vi "Just video2.vi"() -> ()   [LabVIEW 2014]
uses:
  <vilib>/Platform/TimedLoop/XDataNode/wakeup.ctl
  <vilib>/Platform/TimedLoop/XDataNode/XDNodeRunTimeDep.lvlib
  <vilib>/Platform/TimedLoop/XDataNode/nitl_modes.ctl
  <vilib>/Platform/TimedLoop/XDataNode/timing_clust.ctl
  <vilib>/Platform/TimedLoop/XDataNode/XDataNode.xnode
  <vilib>/vision/Avi1.llb/AviRefnum.ctl
panel:
  in  "Image Index":dbl=1.0 min=1.0
  in  "Capture and Save Image":bool
  in  "Averaging":bool
  in  "Reset Averaging":bool
  in  "Capture Video":bool
  out "Image":u32[][](graph)
  in  "New Video File":bool
  in  "Video Index":dbl=1.0 min=1.0 step=1.0
  out "Path Out":path
  in  "Video Capture Rate (Hz)":dbl=30.0
  in  "Stop All":bool
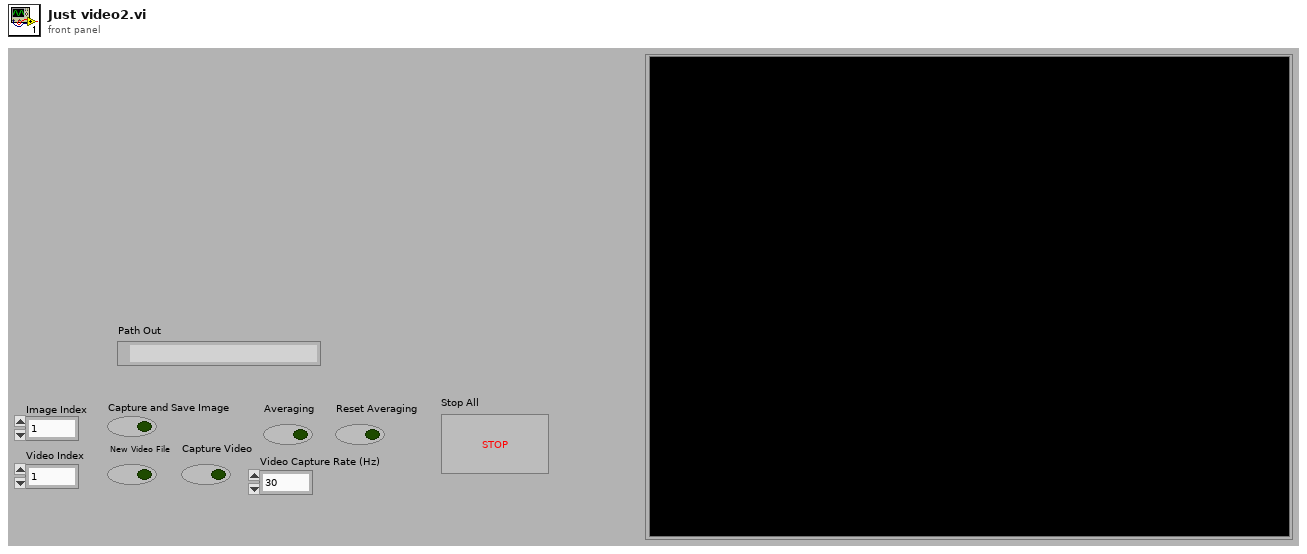
[diagram p1: front panel]
types:
  T1 = enum32{"setting", "request", "request control", "info", "statistics", "system settings", "I/O sub system", "HRT control", "camera descriptions", "device specific data", "event sub system settings", "event sub system results", "image memory manager"}
  T2 = typedef "AviRefnum.ctl" = refnum<k1>
  T3 = typedef "XDNodeRunTimeDep.lvlib/timing_clust.ctl" = cluster{"Expected End [f-1]":u64, "Actual End [f-1]":u64, "Finished Late? [f-1]":bool, "Expected End [i-1]":u64, "Actual End [i-1]":u64, "Finished Late? [i-1]":bool, "Expected Start [i]":u64, "Actual Start [i]":u64, "Expected Start [f]":u64, "Actual Start [f]":u64, "Source Name":string, "Structure Name":string, "Period":i64, "Deadline":i64, "Offset":i64, "Start":i64, "Priority":i32, "Timeout":i32, "Mode":T4, "Wakeup Reason":T5, "Error":errorcluster, "Source Type":string, "Secondary Source Type":string, "Global End Time":u64, "Global Start Time":u64, "Frame Duration":u64, "Iteration Duration":u64, "Assigned CPU":i32, "I/O Scan Engine Mode":u32}
  T4 = typedef "XDNodeRunTimeDep.lvlib/nitl_modes.ctl" = enum32{"No Change", "Process missed periods, maintain original phase", "Discard missed periods, maintain original phase", "Process missed periods, ignore original phase", "Discard missed periods, ignore original phase"}
  T5 = typedef "XDNodeRunTimeDep.lvlib/wakeup.ctl" = enum32{"Normal", "Aborted", "Asynchronous wakeup", "Timing source error", "Timed loop error", "Timeout"}
  T6 = typedef "Image Type" = u32
  T7 = typedef "IMAQ Image.ctl" = refnum<image>
  T8 = typedef "imagedata.ctl" = cluster{"image type":i32, "image depth":i32, "image":u8[], "mask":u8[], "colors":u32[], "Rectangle":cluster{"left":i16, "top":i16, "right":i16, "bottom":i16}}
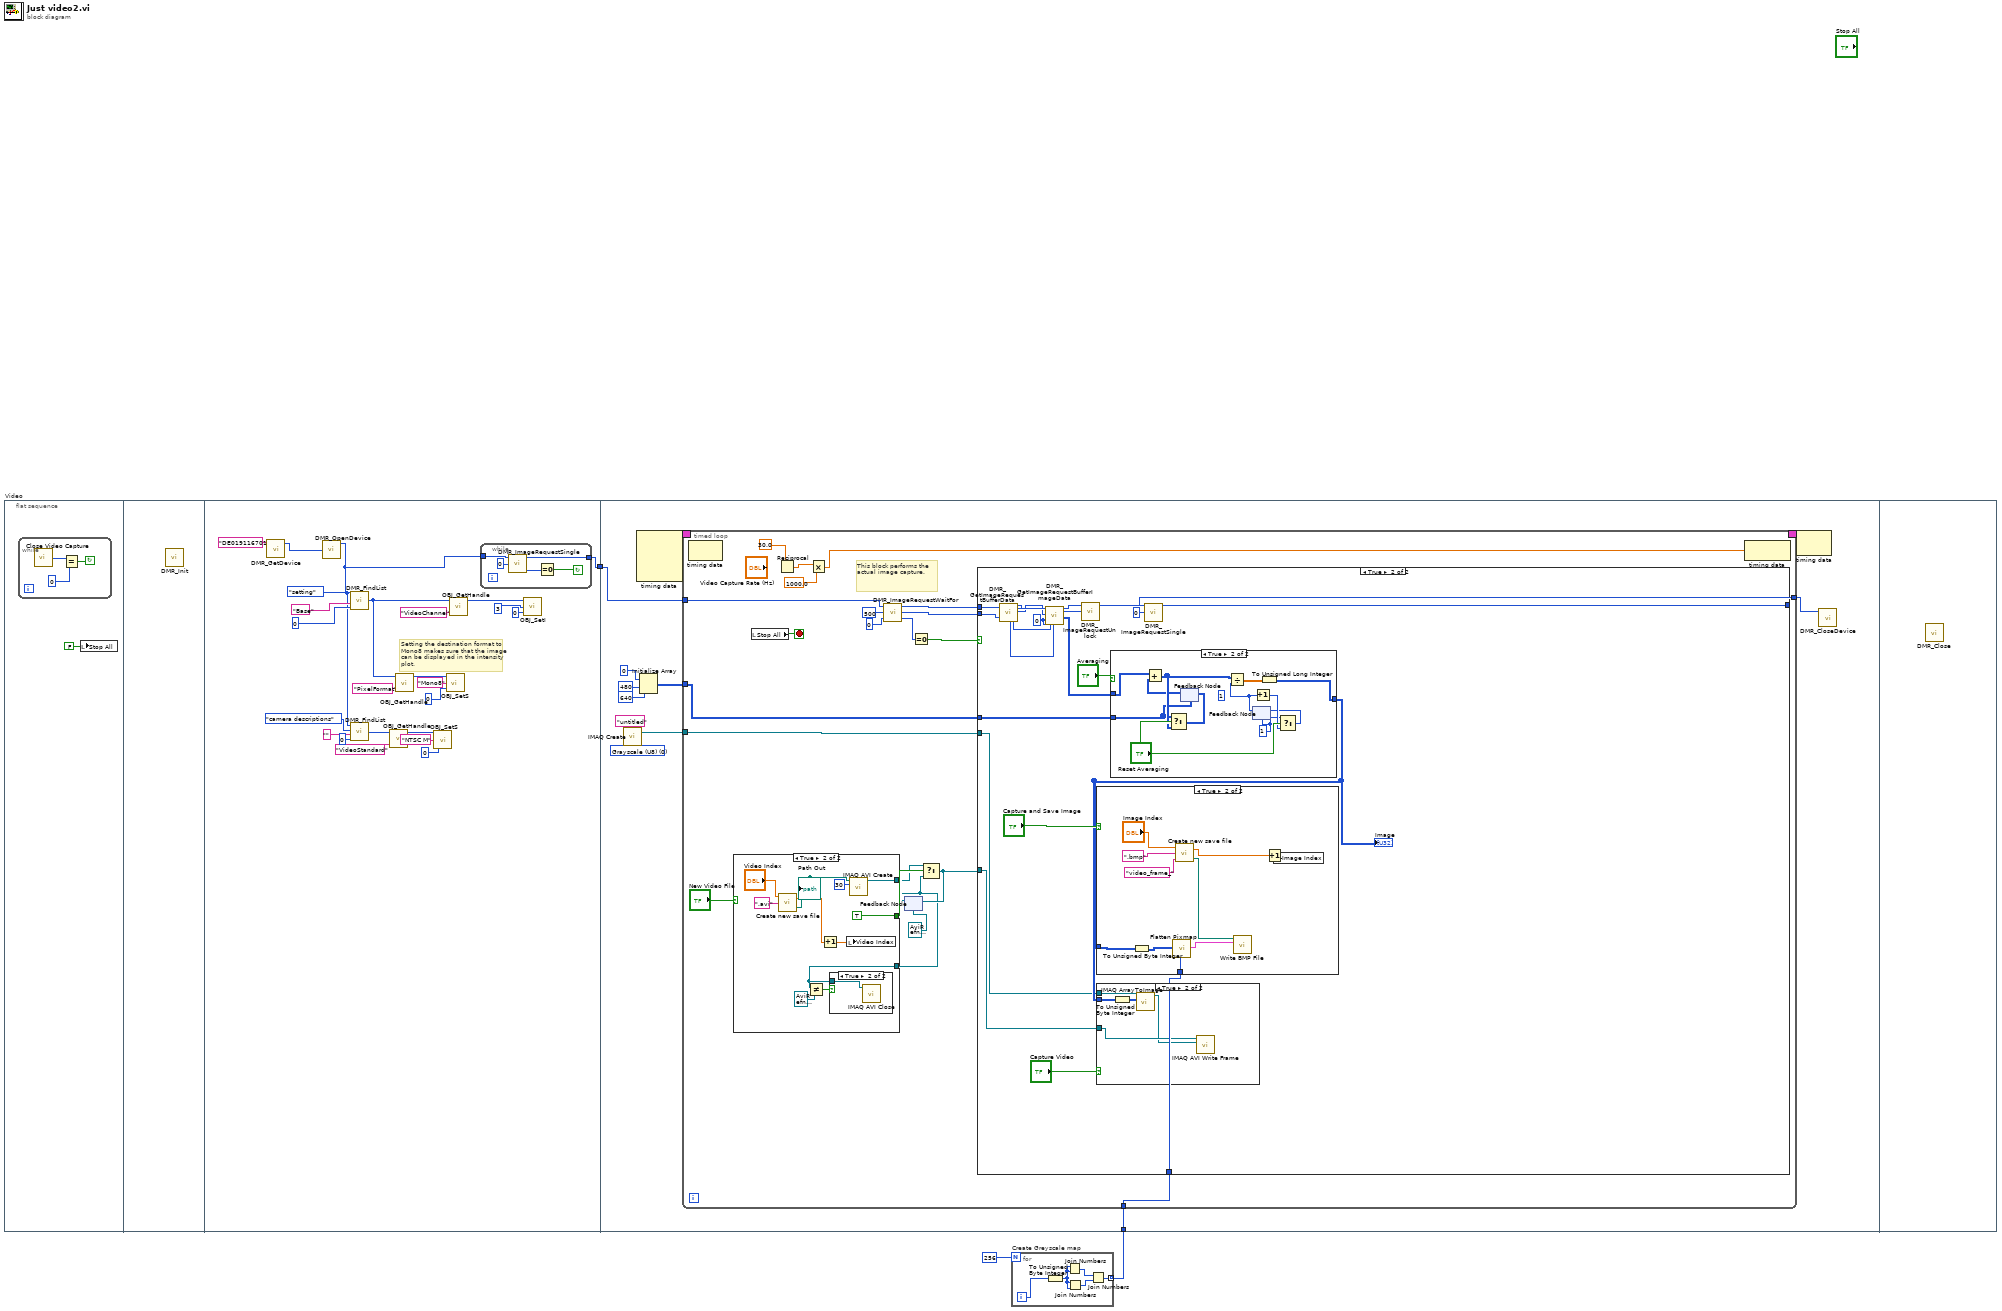
[diagram p0: block diagram]
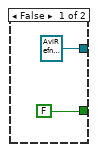
[diagram p2: hidden frame]
diagram:
  n1 = flat-sequence "Video" {
    tunnel: [w12] -> w3
    tunnel: w3 -> [w48]
    tunnel: w1 -> [w46]
    frame #0 {
      n2 = while {
        stop <- w5 continue-if-true
        n3 = call "Close Video Capture.vi"() -> ("error code OUT"=w7:i32)
        n4 = Equal?(x=w7, y=0) -> (x = y?=w5:bool)
      }
      n5 = local write "Stop All"(FALSE ("Stop All")) -> ()
    }
    frame #1 {
      n6 = call "DMR_Init.vi"() -> ()  [unwired: 3 out]
    }
    frame #2 {
      # "Setting the destination format to Mono8 makes sure that the image can be displayed in the intensity plot."
      n7 = call "DMR_GetDevice.vi"("search string IN"="DE019116701") -> ("device handle OUT"=w30:i32)  [unwired: 4 in, 2 out]
      n8 = call "DMR_OpenDevice.vi"("device handle IN"=w30) -> ("driver handle OUT"=w13:i32)  [unwired: 4 out]
      n9 = call "DMR_FindList.vi"("flags IN"=u32 0 ("flags"), "list name IN"="" ("String"), "list type IN"=T1."camera descriptions", "driver handle IN"=w13) -> ("list handle OUT"=w16:i32)  [unwired: 2 out]
      n10 = call "DMR_FindList.vi"("flags IN"=u32 0 ("flags"), "list name IN"="Base", "list type IN"=T1."setting", "driver handle IN"=w13) -> ("list handle OUT"=w14:i32)  [unwired: 2 out]
      n11 = call "OBJ_GetHandle.vi"("object name IN"="VideoStandard", "list handle IN"=w16) -> ("object handle OUT"=w10:i32)  [unwired: 3 out]
      n12 = call "OBJ_GetHandle.vi"("object name IN"="PixelFormat", "list handle IN"=w14) -> ("object handle OUT"=w24:i32)  [unwired: 3 out]
      n13 = call "OBJ_SetS.vi"("value index IN"=0, "value IN"="NTSC M", "object handle IN"=w10) -> ()  [unwired: 2 out]
      n14 = call "OBJ_SetS.vi"("value index IN"=0, "value IN"="Mono8" ("value"), "object handle IN"=w24) -> ()  [unwired: 2 out]
      n15 = call "OBJ_GetHandle.vi"("object name IN"="VideoChannel", "list handle IN"=w14) -> ("object handle OUT"=w20:i32)  [unwired: 3 out]
      n16 = while {
        tunnel: [w35] -> w12
        tunnel: w13 -> [w32]
        stop <- w33 continue-if-true
        n17 = call "DMR_ImageRequestSingle.vi"("request control IN"=0, "driver handle IN"=w32) -> ("error code OUT"=w34:i32, "driver handle OUT"=w35:i32)  [unwired: 2 out]
        n18 = Equal To 0?(x=w34) -> (x = 0?=w33:bool)
      }
      n19 = call "OBJ_SetI.vi"("value index IN"=0, "value IN"=3 ("Video channel"), "object handle IN"=w20) -> ()  [unwired: 2 out]
    }
    frame #3 {
      w43 = T6 0 items=["Grayscale (U8)", "Grayscale (I16)", "Grayscale (SGL)", "Complex (CSG)", "RGB (U32)", "HSL (U32)", "RGB (U64)"] ("Image Type")
      n20 = call "IMAQ Create"("Image Name"="untitled", "Image Type"=w43) -> ("New Image"=w44:T7)  [unwired: 2 in, 2 out]
      n21 = node-c288() -> (w42:T3)  [unwired: 4 out]
      n22 = Initialize Array(u32 0 ("Window Number (0...15)"), 480 ("dimension size"), 640 ("dimension size")) -> (w37:u32[][])
      n23 = timed-loop {
        tunnel: w48 -> [w64]
        tunnel: [w63] -> w47
        tunnel: w46 -> [w62]
        tunnel: w44 -> [w61]
        timing: w42 -> [_]
        timing-out: [_] -> w41
        tunnel: w37 -> [w51]
        stop <- w49 stop-if-true
        # "This block performs the \nactual image capture."
        n24 = node-c288() -> ()  [unwired: 2 out]
        n25 = local read "Stop All"() -> (w49:bool)
        n26 = Reciprocal(x=30.0) -> (1/x=w54:dbl)
        n27 = Multiply(x=w54, y=1000.0) -> (x*y=w52:dbl)
        n28 = call "DMR_ImageRequestWaitFor.vi"("queue number IN"=0, "timeout(ms) IN"=500, "driver handle IN"=w64) -> ("error code OUT"=w68:i32, "request number OUT"=w65:i32, "driver handle OUT"=w66:i32)
        n29 = feedback #1(T2 refnum ("Avi Refnum")) -> (w55:T2)
        n30 = case shown="True" "New Video File" {
          tunnel: [T2 refnum ("Avi Refnum") w85] -> w57
          tunnel: [FALSE TRUE] -> w58
          tunnel: w55 -> [_ w81]
          frame False {
          }
          frame True {
            n31 = call "Create new save file.vi"("Ext"=".avi" ("string"), "Index In"="Video Index") -> ("Path Out"=w77:path, "Index Out"=w78:dbl)  [unwired: 1 in]
            "Path Out" <- w77
            n32 = Not Equal?(x=w81, y=T2 refnum ("Avi Refnum")) -> (x != y?=w82:bool)
            n33 = Increment(x=w78) -> (x+1=w87:dbl)
            n34 = case shown="True" w82 {
              tunnel: w81 -> [_ w88]
              frame False {
              }
              frame True {
                n35 = call "IMAQ AVI Close"("Avi Refnum"=w88) -> ()  [unwired: 1 in, 10 out]
              }
            }
            n36 = local write "Video Index"(w87) -> ()
            n37 = call "IMAQ AVI Create"("Frames Per Second"=u32 30, "AVI Path"=w77) -> ("Avi Refnum"=w85:T2)  [unwired: 5 in, 4 out]
          }
        }
        n38 = Equal To 0?(x=w68) -> (x = 0?=w67:bool)
        n39 = Select(t=w57, s=w58, f=w55) -> (s? t:f=w56:T2)
        n40 = feedback-in #1(w56) -> ()
        n41 = case shown="True" w67 {
          tunnel: w66 -> [w89 w111]
          tunnel: w65 -> [_ w110]
          tunnel: [w89 w107] -> w63
          tunnel: w62 -> [_ w97]
          tunnel: w61 -> [_ w90]
          tunnel: w51 -> [_ w94]
          tunnel: w56 -> [_ w92]
          frame False {
          }
          frame True {
            w101 = u32 0 ("X-offset IN")
            n42 = call "DMR_GetImageRequestBufferData.vi"("driver handle IN"=w111, "request number IN"=w110) -> ("width OUT"=w100:i32, "height OUT"=w99:i32, "driver handle OUT"=w106:i32, "request number OUT"=w105:i32, "bytes per pixel OUT"=w102:i32)  [unwired: 13 out]
            n43 = call "DMR_GetImageRequestBufferImageData.vi"("driver handle IN"=w106, "request number IN"=w105, "bytes per pixel IN"=w102, "X-offset IN"=w101, "Y-offset IN"=w101, "height IN"=w99, "width IN"=w100) -> ("driver handle OUT"=w104:u32, "request number OUT"=w103:u32, "image OUT"=w95:u32[][])  [unwired: 10 out]
            n44 = call "DMR_ImageRequestUnlock.vi"("request number IN"=w103, "driver handle IN"=w104) -> ("driver handle OUT"=w109:i32)  [unwired: 1 in, 2 out]
            n45 = case shown="True" "Averaging" {
              tunnel: w95 -> [w117 w122]
              tunnel: [w117 w121] -> w91
              tunnel: w94 -> [_ w119]
              frame False {
              }
              frame True {
                (unwired) 1
                w127 = 1
                n46 = feedback #2(w119) -> (w118:u32[][])
                n47 = Add(x=w122, y=w118) -> (x+y=w123:u32[][])
                n48 = Select(t=w119, s="Reset Averaging", f=w123) -> (s? t:f=w125:u32[][])
                n49 = feedback-in #2(w125) -> ()
                n50 = feedback #3(w127) -> (w120:i32)
                n51 = Divide(x=w123, y=w120) -> (x/y=w124:dbl[][])
                n52 = Increment(x=w120) -> (x+1=w128:i32)
                n53 = To Unsigned Long Integer(number=w124) -> (unsigned 32bit integer=w121:u32[][])
                n54 = Select(t=w127, s="Reset Averaging", f=w128) -> (s? t:f=w126:i32)
                n55 = feedback-in #3(w126) -> ()
              }
            }
            "Image" <- w91
            n56 = case shown="True" "Capture and Save Image" {
              tunnel: w91 -> [_ w139]
              tunnel: w97 -> [_ w138]
              frame False {
              }
              frame True {
                n57 = To Unsigned Byte Integer(number=w139) -> (unsigned 8bit integer=w135:u8[][])
                n58 = call <vilib>:"Flatten Pixmap.vi"("colors"=w138, "8-bit pixmap"=w135) -> ("image data"=w136:T8)  [unwired: 4 in, 5 out]
                n59 = call "Create new save file.vi"("Insert"="video_frame_" ("string"), "Ext"=".bmp" ("string"), "Index In"="Image Index") -> ("Path Out"=w131:path, "Index Out"=w137:dbl)
                n60 = call <vilib>:"Write BMP File.vi"("image data"=w136, "path to BMP file"=w131) -> ()  [unwired: 1 in, 9 out]
                n61 = Increment(x=w137) -> (x+1=w130:dbl)
                n62 = local write "Image Index"(w130) -> ()
              }
            }
            n63 = case shown="True" "Capture Video" {
              tunnel: w92 -> [_ w116]
              tunnel: w91 -> [_ w114]
              tunnel: w90 -> [_ w113]
              frame False {
              }
              frame True {
                n64 = To Unsigned Byte Integer(number=w114) -> (unsigned 8bit integer=w115:u8[][])
                n65 = call "IMAQ ArrayToImage"("Image Pixels (U8)"=w115, "Image"=w113) -> ("Image Out"=w112:T7)  [unwired: 4 in, 5 out]
                n66 = call "IMAQ AVI Write Frame"("Image"=w112, "Avi Refnum"=w116) -> ()  [unwired: 2 in, 8 out]
              }
            }
            n67 = call "DMR_ImageRequestSingle.vi"("request control IN"=0, "driver handle IN"=w109) -> ("driver handle OUT"=w107:i32)  [unwired: 3 out]
          }
        }
        n68 = node-c288(w52) -> ()  [unwired: 1 out]
      }
      n69 = node-c288(w41) -> ()  [unwired: 1 out]
      n70 = call "DMR_CloseDevice.vi"("driver handle IN"=w47) -> ()  [unwired: 1 in, 4 out]
    }
    frame #4 {
      n71 = call "DMR_Close.vi"() -> ()  [unwired: 1 out]
    }
  }
  n72 = for "Create Greyscale map" {
    N: 256 -> [_]
    tunnel: [w143] -> w1 mode=indexing
    i -> [w146]
    n73 = To Unsigned Byte Integer(number=w146) -> (unsigned 8bit integer=w142:u8)
    n74 = Join Numbers(hi=w142, lo=w142) -> ((hi.lo)=w145:u16)
    n75 = Join Numbers(hi=w142, lo=w142) -> ((hi.lo)=w144:u16)
    n76 = Join Numbers(hi=w145, lo=w144) -> ((hi.lo)=w143:u32)
  }
